vi "close excel file if open.vi"(8 "error in (no error)":errorcluster, 11 "report file path in":path) -> (0 "error out":errorcluster, 3 "report file path out":path)   [LabVIEW 2016]
uses:
  <vilib>/Utility/NIReport.llb/NI_report.lvclass
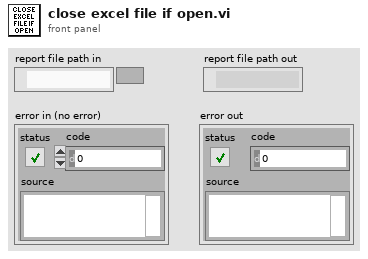
[diagram p1: front panel]
types:
  T1 = enum16{"maximized", "minimized", "normal", "no change"}
  T2 = enum16{"Standard Report", "HTML", "Word", "Excel"}
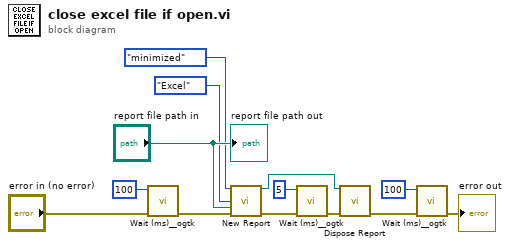
[diagram p0: block diagram]
diagram:
  n1 = call <userlib>:"Wait (ms)__ogtk.vi"("error in (no error)"="error in (no error)", "milliseconds to wait"=u32 100) -> ("error out"=w2:errorcluster)  [unwired: 8 in, 1 out]
  n2 = call <vilib>:"New Report.vi"("window state (normal)"=T1."minimized", "report type"=T2."Excel", "template (empty)"="report file path in", "error in (no error)"=w2) -> ("report out"=w8:refnum<class "NI_report.lvclass">, "error out"=w9:errorcluster)  [unwired: 10 in]
  n3 = call <userlib>:"Wait (ms)__ogtk.vi"("error in (no error)"=w9, "milliseconds to wait"=u32 5) -> ("error out"=w12:errorcluster)  [unwired: 8 in, 1 out]
  n4 = call-dynamic "Dispose Report.vi"("report in"=w8, "error in (no error)"=w12) -> ("error out"=w6:errorcluster)  [unwired: 13 in]
  n5 = call <userlib>:"Wait (ms)__ogtk.vi"("error in (no error)"=w6, "milliseconds to wait"=u32 100) -> ("error out"=→"error out":errorcluster)  [unwired: 8 in, 1 out]
  "report file path out" <- "report file path in"
